vi "Build Spectrum Graph.vi"(0 "Data Cluster":T2) -> (6 "Spectrum Graph":T1(graph))   [LabVIEW 2019, in "Dashboard.lvlib"]
uses:
  Dashboard.lvlib
  Module Data--cluster.ctl
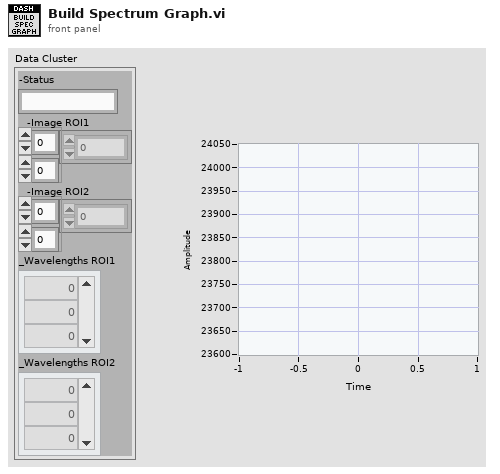
[diagram p1: front panel]
types:
  T1 = cluster{"Ramp Pattern":dbl[], "Image ROI1":u16[]}[]
  T2 = typedef "Dashboard.lvlib/Module Data--cluster.ctl" = cluster{"-Status":string, "-Image ROI1":u16[][], "-Image ROI2":u16[][], "_Wavelengths ROI1":dbl[], "_Wavelengths ROI2":dbl[]}
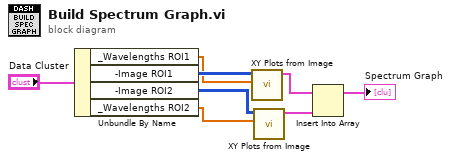
[diagram p0: block diagram]
diagram:
  n1 = Unbundle By Name("Data Cluster") -> ("_Wavelengths ROI1"=w2:dbl[], "-Image ROI1"=w7:u16[][], "-Image ROI2"=w6:u16[][], "_Wavelengths ROI2"=w1:dbl[])
  n2 = call "XY Plots from Image.vi"("wavelengths"=w2, "Image ROI1"=w7) -> ("Array"=w5:T1)  [unwired: 9 in]
  n3 = call "XY Plots from Image.vi"("wavelengths"=w1, "Image ROI1"=w6) -> ("Array"=w4:T1)  [unwired: 9 in]
  n4 = Insert Into Array(array=w5, new element=w4) -> (→"Spectrum Graph":T1)  [unwired: 1 in]
